vi "myRMS.vi"(10 "LptRMS":i32, 11 "dane":dbl[](array[numeric])) -> (3 "rms_sign":dbl[](array[numeric]))   [LabVIEW 2020]
uses:
  <vilib>/Analysis/5stat.llb/RMS (DBL).vi
  <vilib>/Analysis/NI_AALPro.lvlib
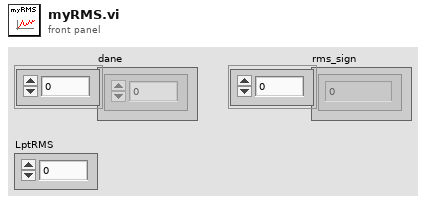
[diagram p1: front panel]
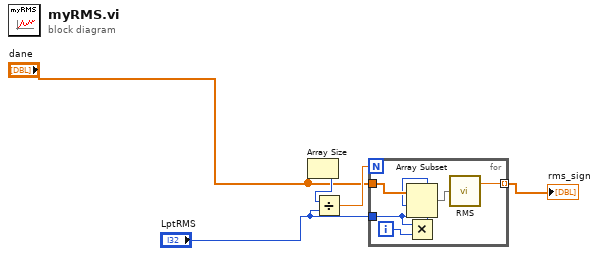
[diagram p0: block diagram]
diagram:
  n1 = Array Size(array="dane") -> (size(s)=w3:i32)
  n2 = Divide(x=w3, y="LptRMS") -> (x/y=w5:dbl)
  n3 = for {
    N: w5 -> [_]
    tunnel: "dane" -> [w11]
    tunnel: "LptRMS" -> [w9]
    tunnel: [w6] -> w1 mode=indexing
    i -> [w10]
    n4 = Multiply(x=w9, y=w10) -> (x*y=w8:i32)
    n5 = Array Subset(array=w11, index=w8, length=w9) -> (w7:dbl[])
    n6 = call-poly <vilib>:"RMS.vi"("X"=w7) -> ("rms value"=w6:dbl)  [unwired: 1 out]
  }
  "rms_sign" <- w1
